vi "peirce_method.vi"(2 "DesvioPadrão":dbl, 3 "DesviosAbsolutos":dbl[](array[numeric])=[20.0, 20.1, 19.9, 20.2, 25.0, 20.0, 20.2, 20.1]) -> (0 "IndexRemovidos":i32[](array[numeric]), 1 "PeirceTol":dbl)   [LabVIEW 2016]
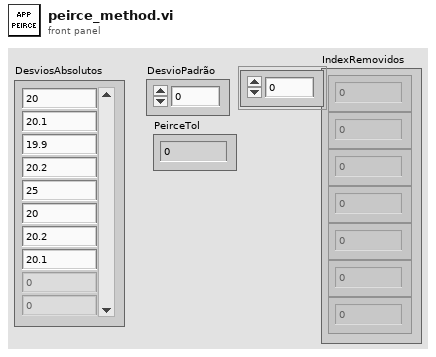
[diagram p1: front panel]
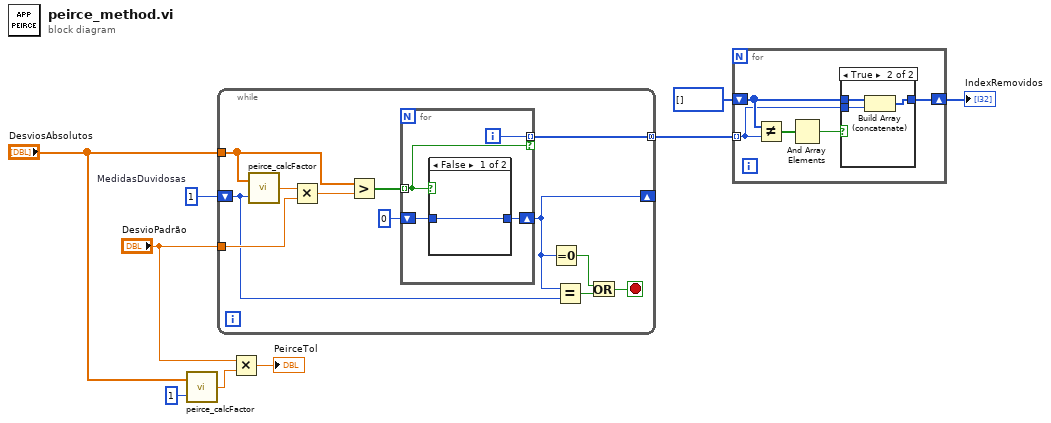
[diagram p0: block diagram]
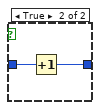
[diagram p3: hidden frame]
diagram:
  w9 = 1  # MedidasDuvidosas
  n1 = call "peirce_calcFactor.vi"("n"=1, "DesviosAbsolutos"="DesviosAbsolutos") -> ("x"=w3:dbl)
  n2 = while {
    shift-right: [w13] -> _
    shift-left: w9 -> [w16]
    tunnel: "DesvioPadrão" -> [w21]
    tunnel: "DesviosAbsolutos" -> [w15]
    tunnel: [w14] -> w8 mode=concatenating
    stop <- w10 stop-if-true
    n3 = call "peirce_calcFactor.vi"("n"=w16, "DesviosAbsolutos"=w15) -> ("x"=w20:dbl)
    n4 = Multiply(x=w20, y=w21) -> (x*y=w19:dbl)
    n5 = Greater?(x=w15, y=w19) -> (0:w18:bool[])
    n6 = for {
      tunnel: w18 -> [w22] mode=indexing
      shift-right: [w24] -> w13
      shift-left: 0 -> [w25]
      tunnel: [w23] -> w14 mode=indexing if=w22
      i -> [w23]
      n7 = case shown="False" w22 {
        tunnel: w25 -> [w26 w28]
        tunnel: [w26 w27] -> w24
        frame False {
        }
        frame True {
          n8 = Increment(x=w28) -> (x+1=w27:i32)
        }
      }
    }
    n9 = Equal To 0?(x=w13) -> (x = 0?=w11:bool)
    n10 = Equal?(x=w13, y=w16) -> (x = y?=w12:bool)
    n11 = Or(x=w11, y=w12) -> (x .or. y?=w10:bool)
  }
  n12 = Multiply(x="DesvioPadrão", y=w3) -> (x*y=→"PeirceTol":dbl)
  n13 = for {
    tunnel: w8 -> [w31] mode=indexing
    shift-right: [w29] -> w6
    shift-left: i32[] [] -> [w32]
    n14 = Not Equal?(x=w32, y=w31) -> (x != y?=w33:bool[])
    n15 = And Array Elements(Boolean array=w33) -> (logical AND=w30:bool)
    n16 = case shown="True" w30 {
      tunnel: w32 -> [w34 w37]
      tunnel: w31 -> [_ w36]
      tunnel: [w34 w35] -> w29
      frame False {
      }
      frame True {
        n17 = Build Array (concatenate)(w37, w36) -> (w35:i32[])
      }
    }
  }
  "IndexRemovidos" <- w6
